vi "Open and Disable Source Separation (VI).vi"(8 "Error In":errorcluster, 11 "VI Path":path) -> (0 "Error Out":errorcluster)   [LabVIEW 2014]
doc: "Copyright (c) 2018 Sze Howe Koh\n\nThis Source Code Form is subject to the terms of the Mozilla Public License, v. 2.0. If a copy of the MPL was not distributed with this file, You can obtain one at http://mozilla.org/MPL/2.0/."
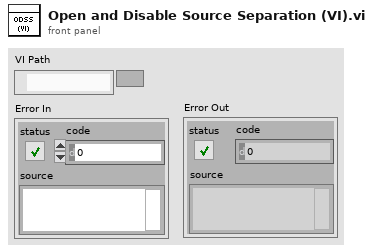
[diagram p1: front panel]
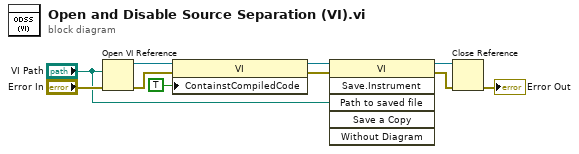
[diagram p0: block diagram]
diagram:
  n1 = Open VI Reference(vi path="VI Path", error in (no error)="Error In") -> (vi reference=w9:refnum<vi>, error out=w4:errorcluster)  [unwired: 4 in]
  n2 = property class="VI"(reference=w9, error in=w4, "ContainstCompiledCode"=TRUE ("Contains Compiled Code")) -> (reference out=w7:refnum<vi>, error out=w3:errorcluster)
  n3 = invoke class="VI" method="Save.Instrument"(reference=w7, error in=w3, "Path to saved file"="VI Path") -> (reference out=w5:refnum<vi>, error out=w2:errorcluster)  [unwired: 3 in, 4 out]
  n4 = Close Reference(reference=w5, error in (no error)=w2) -> (error out=→"Error Out":errorcluster)
